vi "Measure.vi"(8 "error in (no error)":errorcluster, 11 "Hardware in":refnum<class "Mag Lab Hardware.lvclass">) -> (0 "error out":errorcluster, 3 "Hardware out":refnum<class "Mag Lab Hardware.lvclass">)   [LabVIEW 2015, in "Mag Lab Hardware.lvclass"]
uses:
  Mag Lab Hardware.lvclass
  Mag Lab Hardware.lvclass/Mag Lab Hardware.ctl
  Mag Lab Measure Controller Messages/Recieve Result Msg/Recieve Result Msg.lvclass/Recieve Result Msg.ctl
  <vilib>/ActorFramework/Message Enqueuer/Message Enqueuer.lvclass/Message Enqueuer.ctl
  <vilib>/ActorFramework/Message Enqueuer/Enqueue.vi
  <vilib>/ActorFramework/Message Priority Queue/Priority Enqueue.vi
  <vilib>/ActorFramework/Message Enqueuer/Message Enqueuer.lvclass
  Mag Lab Measure Controller Messages/Recieve Result Msg/Recieve Result Msg.lvclass
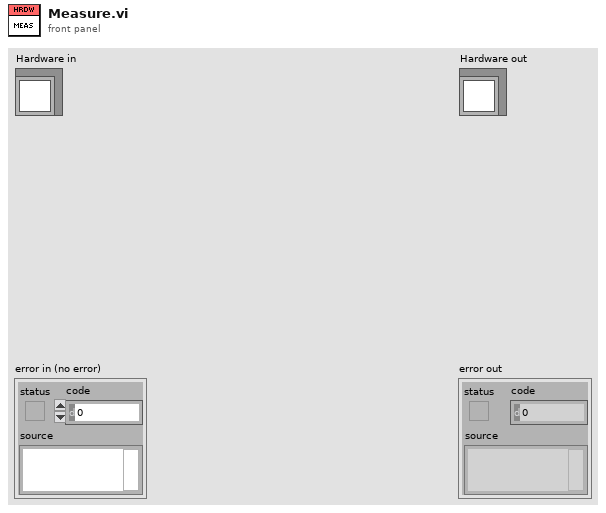
[diagram p1: front panel]
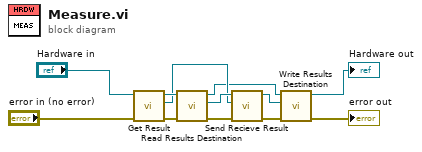
[diagram p0: block diagram]
diagram:
  n1 = call-dynamic "Get Result.vi"("error in (no error)"="error in (no error)", "Mag Lab Hardware in"="Hardware in") -> ("error out"=w3:errorcluster, "Mag Lab Result.lvclass"=w6:refnum<class "Mag Lab Result.lvclass">, "Mag Lab Hardware out"=w8:refnum<class "Mag Lab Hardware.lvclass">)  [unwired: 7 in]
  n2 = call "Read Results Destination.vi"("error in (no error)"=w3, "Mag Lab Hardware in"=w8) -> ("error out"=w2:errorcluster, "Actor Framework:Message Enqueuer"=w7:refnum<class "Message Enqueuer.lvclass">, "Mag Lab Hardware out"=w5:refnum<class "Mag Lab Hardware.lvclass">)  [unwired: 7 in]
  n3 = call "Send Recieve Result.vi"("error in (no error)"=w2, "Mag Lab Result.lvclass"=w6, "Message Enqueuer"=w7) -> ("error out"=w1:errorcluster, "Message Enqueuer out"=w4:refnum<class "Message Enqueuer.lvclass">)  [unwired: 7 in]
  n4 = call "Write Results Destination.vi"("error in (no error)"=w1, "Actor Framework:Message Enqueuer"=w4, "Mag Lab Hardware in"=w5) -> ("error out"=→"error out":errorcluster, "Mag Lab Hardware out"=→"Hardware out":refnum<class "Mag Lab Hardware.lvclass">)  [unwired: 7 in]
